vi "CTRE_Phoenix_MotorControl_BufferedTrajectoryPointStream_Open.vi"(8 "error in":errorcluster) -> (0 "error out":errorcluster, 3 "BufferedTrajectoryPointStream_DevRef":T1)   [LabVIEW 2019]
uses:
  <vilib>/Rock Robotics/WPI/ThirdParty/Phoenix-LabVIEW/Motor Controller/Controls/CTRE_Phoenix_MotorControl_BufferedTrajectoryPointStream_DeviceRef.ctl
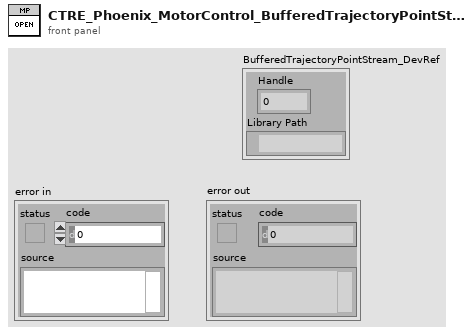
[diagram p1: front panel]
types:
  T1 = typedef "CTRE_Phoenix_MotorControl_BufferedTrajectoryPointStream_DeviceRef.ctl" = cluster{"Handle":u64, "Library Path":path}
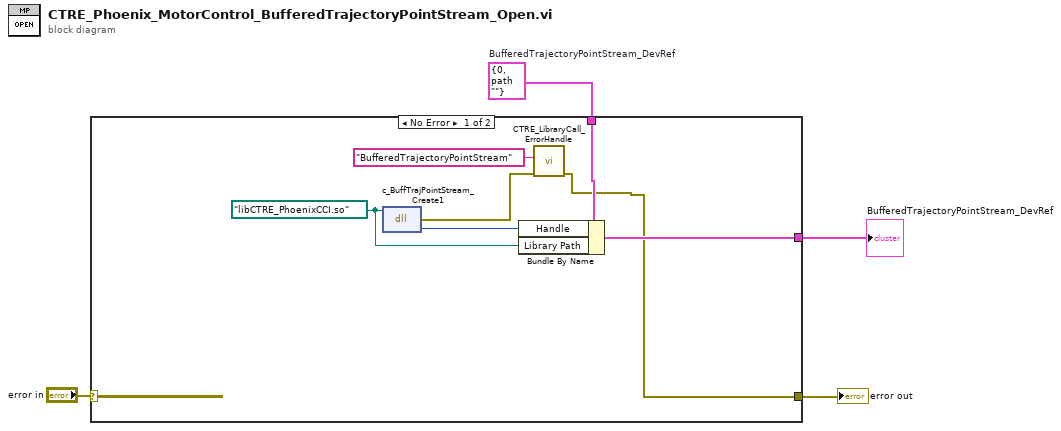
[diagram p0: block diagram]
diagram:
  w2 = T1 {"Handle"=0, "Library Path"=path ""}  # BufferedTrajectoryPointStream_DevRef
  n1 = case shown="No Error" "error in" {
    selector: "error in" -> [_ w12]
    tunnel: [w6 w12] -> w3
    tunnel: w2 -> [w11 _]
    tunnel: [w9 _] -> w1
    frame No Error {
      w10 = path "libCTRE_PhoenixCCI.so" ("path in")
      n2 = dll-call lib="?" fn="c_BuffTrajPointStream_Create1"(path in=w10) -> (error out=w8:errorcluster, "handle"=w5:u64)  [unwired: 2 in, 1 out]
      n3 = Bundle By Name(cluster=w11, "Handle"=w5, "Library Path"=w10) -> (w9:T1)
      n4 = call <vilib>:"CTRE_LibraryCall_ErrorHandle.vi"("error in"=w8, "DeviceType"="BufferedTrajectoryPointStream") -> ("error out"=w6:errorcluster)  [unwired: 9 in]
    }
    frame Error {
    }
  }
  "error out" <- w3
  "BufferedTrajectoryPointStream_DevRef" <- w1
